vi "Actor Core.vi"(8 "error in":errorcluster, 11 "RandomDataChart in":refnum<class "ActorAutoRegPanel.lvclass">) -> (0 "error out":errorcluster, 3 "Actor out":refnum<class "Actor.lvclass">)   [LabVIEW 2015, in "TestViewables.lvlib" / "ActorAutoRegPanel.lvclass"]
doc: "(<B>Filename</B>: Actor Framework.lvlib:Actor.lvclass:Actor Core.vi)\n\nReceives messages to the actor, reacts to them, and initiates any error handling that may shut the actor down.\n\nDescendant classes may override this VI to append parallel tasks for the actor to complete while it handles messages. Overrides use the Call Parent Method node.\n\n<License>\nCopyright © 2017 Composed Systems, LLC | All rights reserved\nwww.composed.io\n\nAuthor: Ethan Stern <ethan.stern@composed.io>\n\nThis software is provided \"AS IS\" WITHOUT WARRANTIES, either express or implied, AND IS FOR EDUCATIONAL PURPOSES ONLY.\n</License>"
uses:
  ActorAutoRegPanel.lvclass
  <vilib>/ActorFramework/Actor/Actor.lvclass
  <vilib>/ActorFramework/Actor/Actor.lvclass/Actor.ctl
  <vilib>/ActorFramework/Message Enqueuer/Message Enqueuer.lvclass/Message Enqueuer.ctl
  Framework/AutoRegistration/ActorAutoRegistration/ActorAutoRegistration.lvclass/ActorAutoRegistration.ctl
  <vilib>/ActorFramework/Message Enqueuer/Init from Existing Queue.vi
  Framework/AutoRegistration/AutoRegistration/Register for Panel Events.vi
  Framework/IViewable/IViewable/IViewable.lvclass
  <vilib>/ActorFramework/Message Enqueuer/Message Enqueuer.lvclass
  Framework/AutoRegistration/ActorAutoRegistration/ActorAutoRegistration.lvclass
  Framework/IObserver/IObserver/IObserver.lvclass
panel:
  out "Cluster":T1
  in  "DBL":dbl
  in  "I32":i32
  in  "Whitaker":bool caption="Latch When Released"
  in  "Walton":bool caption="Latch Until Released"
  in  "Launch Dialog":bool
  in  "Guthrie":bool caption="Switch Until Released"
  in  "Harrelson":bool caption="Switch When Released"
  in  "Gump":bool caption="Latch When Pressed"
  in  "Wilson":bool caption="Switch When Pressed"
  # "An actor implementing\nfull auto-registration"
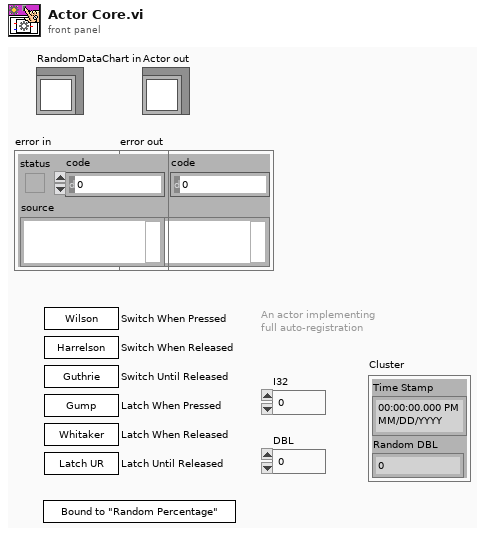
[diagram p1: front panel]
types:
  T1 = cluster{"Time Stamp":timestamp, "Random DBL":dbl}
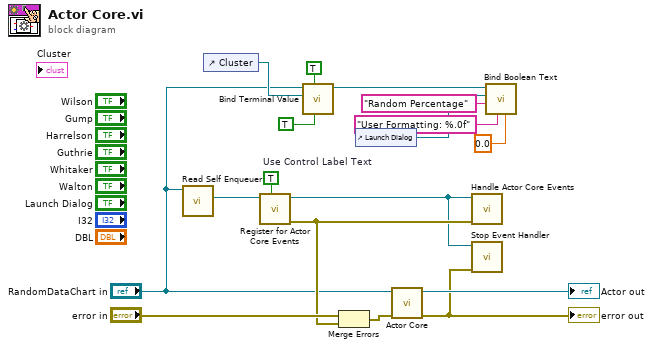
[diagram p0: block diagram]
diagram:
  w10 = TRUE  # Use Control Label Text
  n1 = call <vilib>:"Read Self Enqueuer.vi"("Actor"="RandomDataChart in") -> ("Self Enqueuer"=w14:refnum<class "Message Enqueuer.lvclass">)  [unwired: 10 in]
  n2 = control-ref of="Cluster"() -> (w9:refnum<vi>)
  n3 = call "Register for Actor Core Events.vi"("Use Label Text (F=Use Caption)"=w10, "Actor Enqueuer"=w14) -> ("error out"=w12:errorcluster, "ActorAutoRegistration Out"=w11:refnum<class "ActorAutoRegistration.lvclass">)  [unwired: 8 in]
  n4 = call "Bind Terminal Value.vi"("Value Changes Only? (T)"=TRUE ("Value Changes Only? (F)"), "Bind by Label (F=Bind by Caption)"=TRUE ("Use Label Text (F=Use Caption)"), "Ctl Refnum"=w9, "IObserver in"="RandomDataChart in") -> ("IObserver out"=w5:refnum<class "ActorAutoRegPanel.lvclass">)  [unwired: 6 in, 1 out]
  n5 = Merge Errors("error in", w12) -> (w15:errorcluster)
  n6 = control-ref of="Launch Dialog"() -> (w4:refnum<vi>)
  n7 = call-parent "Actor Core.vi"("error in"=w15, "IViewable In"="RandomDataChart in") -> ("error out"=w13:errorcluster, "Actor out"=→"Actor out":refnum<class "Actor.lvclass">)  [unwired: 8 in]
  "error out" <- w13
  n8 = call-dynamic "Handle Actor Core Events.vi"("error in (no error)"=w12, "ActorAutoRegistration"=w11) -> ()  [unwired: 9 in, 1 out]
  n9 = call-dynamic "Stop Event Handler.vi"("error in (no error)"=w13, "ActorAutoRegistration In"=w11) -> ()  [unwired: 9 in, 1 out]
  n10 = call "Bind Boolean Text.vi"("Data Type"=0.0, "Format String"="User Formatting: %.0f", "Topic Name (Use Control Text)"="Random Percentage", "Bool Refnum"=w4, "IObserver in"=w5) -> ()  [unwired: 5 in, 2 out]
